vi "Clear All Errors.vi"(0 "error in (no error)":errorcluster) -> (2 "error out":errorcluster)   [LabVIEW 2019]
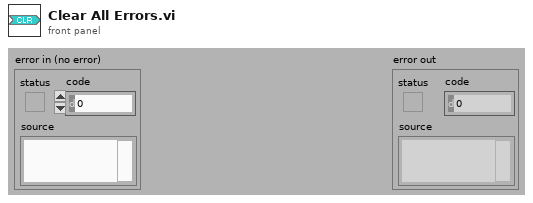
[diagram p1: front panel]
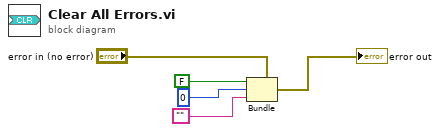
[diagram p0: block diagram]
diagram:
  n1 = Bundle(cluster="error in (no error)", "status"=FALSE, "code"=0, "source"="") -> (→"error out":errorcluster)
